vi "4p1_HW_Task1_fishele.vi"() -> ()   [LabVIEW 2021]
uses:
  <vilib>/express/express arith-compare/Formula/XNode/ExpressFormulaBlockNode.xnode
panel:
  out "Final Result in ft":dbl
  out "Angle 3 in deg":dbl
  out "Length 3":dbl
  out "Length 2":dbl
  out "Length 1":dbl
  out "Angle 1 in deg":dbl
  out "Angle 2 in deg":dbl
  in  "Perpendicular distance of fish from the inner wall":dbl=1.0
  in  "Perpendicular distance from the person to the outer wall of the tank":dbl=2.0
  in  "Wall thickness":dbl=0.5
  in  "Refractive index of the water":dbl=1.33
  in  "Refractive index of the glass":dbl=1.69
  in  "Refractive index of air":dbl=1.0
  in  "Height above eye level":dbl=1.0
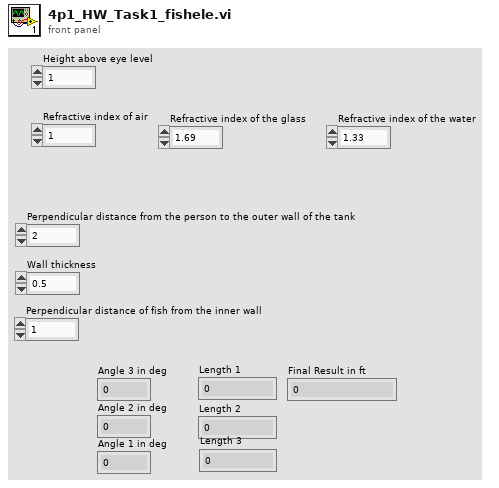
[diagram p1: front panel]
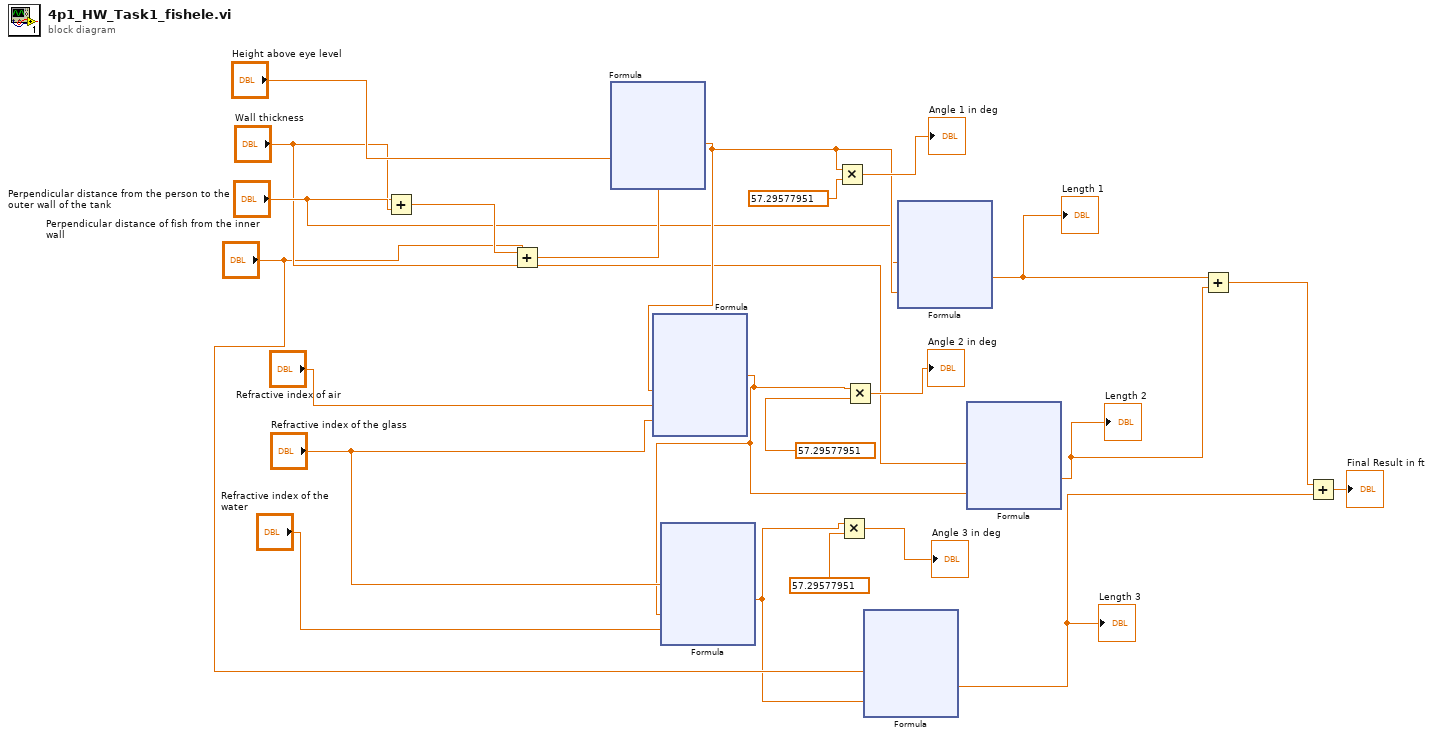
[diagram p0: block diagram]
diagram:
  n1 = Add(x="Wall thickness", y="Perpendicular distance from the person to the outer wall of the tank") -> (x+y=w22:dbl)
  n2 = Add(x=w22, y="Perpendicular distance of fish from the inner wall") -> (x+y=w21:dbl)
  n3 = xnode "Formula"("h"="Height above eye level", "d"=w21) -> ("Result"=w13:dbl)  [unwired: 1 in, 1 out]
  n4 = xnode "Formula"("angle1"=w13, "RIA"="Refractive index of air", "RIG"="Refractive index of the glass") -> ("Result"=w11:dbl)  [unwired: 1 in, 1 out]
  n5 = xnode "Formula"("RIG"="Refractive index of the glass", "angle2"=w11, "RIW"="Refractive index of the water") -> ("Result"=w8:dbl)  [unwired: 1 in, 1 out]
  n6 = Multiply(x=w13, y=57.29577951) -> (x*y=→"Angle 1 in deg":dbl)
  n7 = Multiply(x=w8, y=57.29577951) -> (x*y=→"Angle 3 in deg":dbl)
  n8 = Multiply(x=w11, y=57.29577951) -> (x*y=→"Angle 2 in deg":dbl)
  n9 = xnode "Formula"("DTF"="Perpendicular distance of fish from the inner wall", "angle3"=w8) -> ("Result"=w3:dbl)  [unwired: 1 in, 1 out]
  "Length 3" <- w3
  n10 = xnode "Formula"("DTT"="Perpendicular distance from the person to the outer wall of the tank", "angle1"=w13) -> ("Result"=w4:dbl)  [unwired: 1 in, 1 out]
  "Length 1" <- w4
  n11 = xnode "Formula"("THCK"="Wall thickness", "angle2"=w11) -> ("Result"=w5:dbl)  [unwired: 1 in, 1 out]
  "Length 2" <- w5
  n12 = Add(x=w4, y=w5) -> (x+y=w2:dbl)
  n13 = Add(x=w2, y=w3) -> (x+y=→"Final Result in ft":dbl)
